vi "Convert Selected Column to Actual Message Log Column.vi"(10 "Visible ML Columns":bool[](array[boolean]), 11 "Selected Column":i32=1) -> (3 "Actual Column":i32)   [LabVIEW 2017, in "Message Log.lvclass"]
uses:
  Message Log.lvclass
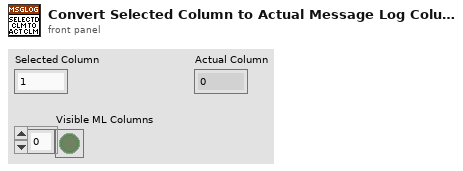
[diagram p1: front panel]
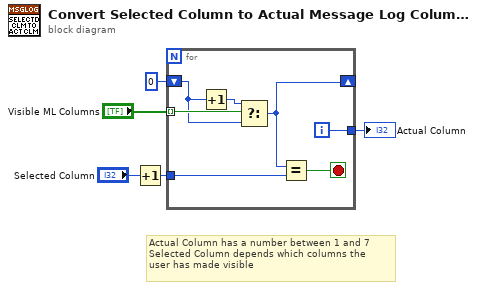
[diagram p0: block diagram]
diagram:
  # "Actual Column has a number between 1 and 7\nSelected Column depends which columns the \nuser has made visible"
  n1 = Increment(x="Selected Column") -> (x+1=w4:i32)
  n2 = for {
    tunnel: "Visible ML Columns" -> [w12] mode=indexing
    shift-right: [w8] -> _
    shift-left: 0 -> [w10]
    tunnel: w4 -> [w9]
    tunnel: [w6] -> w3
    i -> [w6]
    stop <- w7 stop-if-true
    n3 = Increment(x=w10) -> (x+1=w11:i32)
    n4 = Select(t=w11, s=w12, f=w10) -> (s? t:f=w8:i32)
    n5 = Equal?(x=w8, y=w9) -> (x = y?=w7:bool)
  }
  "Actual Column" <- w3
